vi "Logging Error.vi"(8 "error in (no error)":errorcluster, 10 "Log Data":T1, 11 "Elevator Controller Actor in":refnum<class "Elevator Controller Actor.lvclass">) -> (0 "error out":errorcluster, 3 "Elevator Controller Actor out":refnum<class "Elevator Controller Actor.lvclass">)   [LabVIEW 2022 SP3, in "Elevator Controller Actor.lvlib" / "Elevator Controller Actor.lvclass"]
uses:
  Elevator Controller Actor.lvclass
  Elevator Controller Actor.lvclass/Elevator Controller Actor.ctl
  Error Level.ctl
  Log Data.ctl
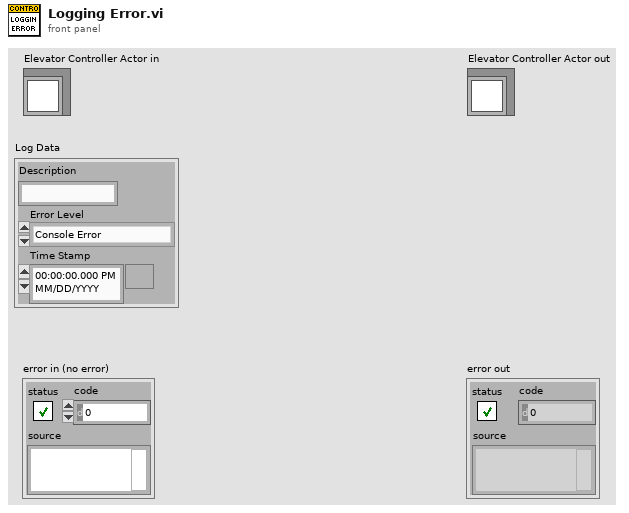
[diagram p1: front panel]
types:
  T1 = typedef "Elevator Controller Actor.lvlib/Elevator Controller Actor.lvclass/Log Data.ctl" = cluster{"Description":string, "Error Level":T2, "Time Stamp":timestamp}
  T2 = typedef "Elevator Controller Actor.lvlib/Elevator Controller Actor.lvclass/Error Level.ctl" = enum16{"Console Error", "Sensor Interface IO Error", "Process Step Error"}
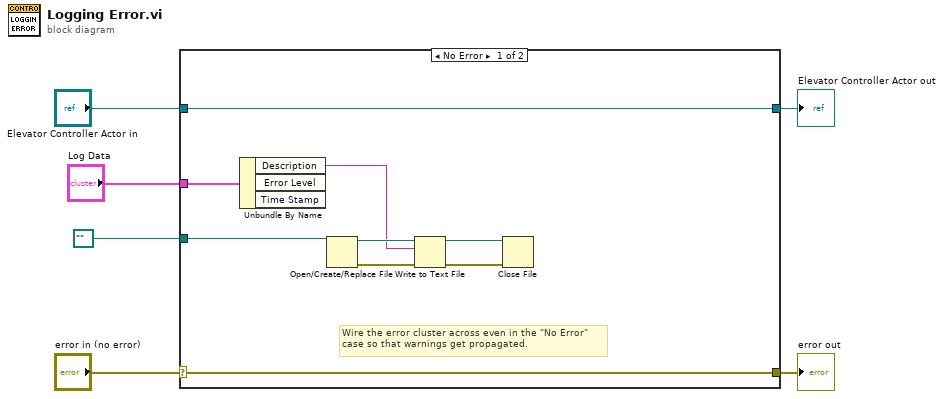
[diagram p0: block diagram]
diagram:
  n1 = case shown="No Error" "error in (no error)" {
    selector: "error in (no error)" -> [w14 w17]
    tunnel: [w14 w17] -> w5
    tunnel: [w15 w16] -> w3
    tunnel: "Elevator Controller Actor in" -> [w15 w16]
    tunnel: "Log Data" -> [w9 _]
    tunnel: path "" ("file path (use dialog)") -> [w7 _]
    frame No Error {
      # "Wire the error cluster across even in the \"No Error\"\ncase so that warnings get propagated."
      n2 = Unbundle By Name(w9) -> ("Description"=w8:string)  [unwired: 2 out]
      n3 = Open/Create/Replace File(file path (use dialog)=w7) -> (refnum out=w11:refnum<file>, error out=w13:errorcluster)  [unwired: 5 in, 1 out]
      n4 = Write to Text File(file (use dialog)=w11, text=w8, error in=w13) -> (refnum out=w10:refnum<file>, error out=w12:errorcluster)  [unwired: 1 in, 1 out]
      n5 = Close File(refnum=w10, error in=w12) -> ()  [unwired: 2 out]
    }
    frame Error {
    }
  }
  "error out" <- w5
  "Elevator Controller Actor out" <- w3
